vi "EnableCache VxWorks.vi"(8 "error in (no error)":errorcluster, 11 "Cache Type":enum16{"_INSTRUCTION_CACHE", "_DATA_CACHE"}(ring)) -> (0 "error out":errorcluster, 3 "Status":u32)   [LabVIEW 2014]
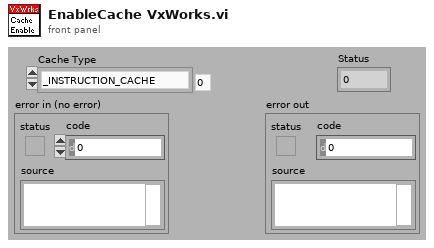
[diagram p1: front panel]
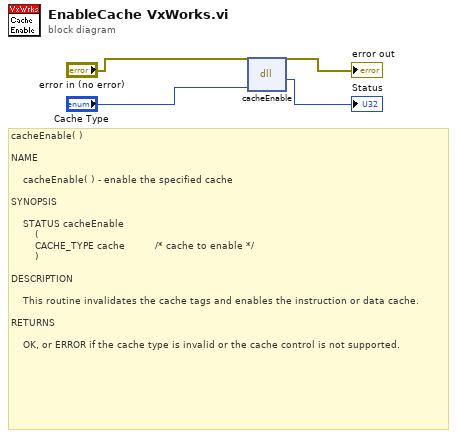
[diagram p0: block diagram]
diagram:
  # "cacheEnable( )\n\nNAME\n\n    cacheEnable( ) - enable the specified cache\n\nSYNOPSIS\n\n    STATUS cacheEnable\n        (\n        CACHE_TYPE cache          /* cache to enable */\n        )\n\nDESCRIPTION\n\n    This routine invalidates the cache tags and enables the instruction or data cache.\n\nRETURNS\n\n    OK, or ERROR if the cache type is invalid or the cache control is not supported."
  n1 = dll-call lib="LabVIEW" fn="cacheEnable" ("vxWorks:cacheInvalidate")("Cache_Type"="Cache Type") -> ("Status"=→"Status":u32)  [unwired: 4 in, 2 out]
  "error out" <- "error in (no error)"
